vi "Sampling Frequency.vi"() -> (0 "Sampling Frequency":dbl)   [LabVIEW 2013]
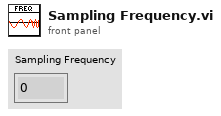
[diagram p1: front panel]
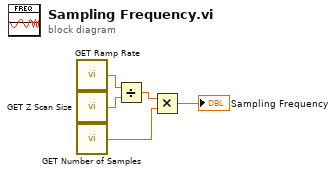
[diagram p0: block diagram]
diagram:
  n1 = call "GET Ramp Rate.vi"() -> ("Ramp Rate"=w4:dbl)
  n2 = call "GET Z Scan Size.vi"() -> ("Z Scan Size"=w5:dbl)
  n3 = call "GET Number of Samples.vi"() -> ("Number of Samples"=w2:dbl)
  n4 = Divide(x=w4, y=w5) -> (x/y=w3:dbl)
  n5 = Multiply(x=w3, y=w2) -> (x*y=→"Sampling Frequency":dbl)
